vi "math.vi"() -> ()   [LabVIEW 2012]
panel:
  out "Waveform Graph":dbl[](graph)
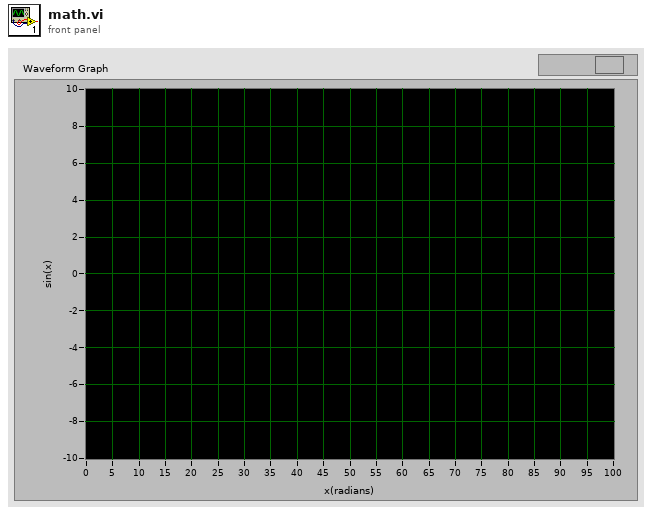
[diagram p1: front panel]
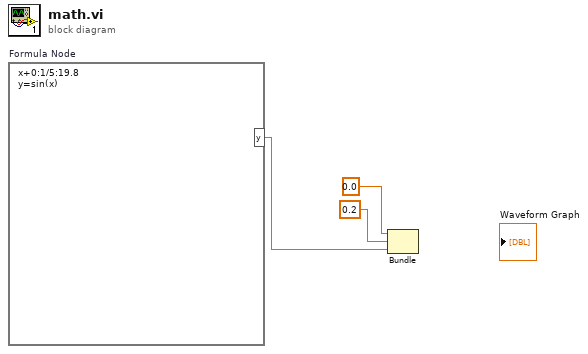
[diagram p0: block diagram]
diagram:
  n1 = formula code="x+0:1/5:19.8\ny=sin(x)"() -> ("y"=w1:dbl)
  n2 = Bundle(0.0, 0.2, "y"=w1) -> ()  [unwired: 1 in, 1 out]
